vi "Threshold Filter.vi"(11 "Image In":T1) -> (3 "Image Out":T1)   [LabVIEW 2011]
uses:
  <vilib>/vision/Image Controls.llb/IMAQ Image.ctl
  <vilib>/vision/NI_Vision_Development_Module.lvlib
panel:
  in  "Replace Value":i32=1
  out "ThreshHold Filter":T1(plugin-control)
  in  "Blue or Luma or Val or Inten Range":cluster{"Lower value":i32, "Upper value":i32}={"Lower value"=0, "Upper value"=255}
  in  "Green or Sat Range":cluster{"Lower value":i32, "Upper value":i32}={"Lower value"=0, "Upper value"=255}
  in  "Red or Hue Range":cluster{"Lower value":i32, "Upper value":i32}={"Lower value"=0, "Upper value"=255}
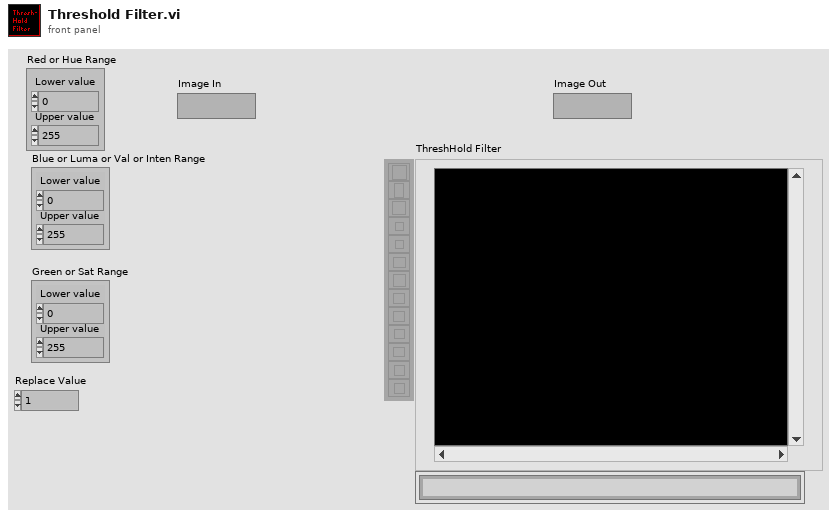
[diagram p1: front panel]
types:
  T1 = typedef "IMAQ Image.ctl" = refnum<image>
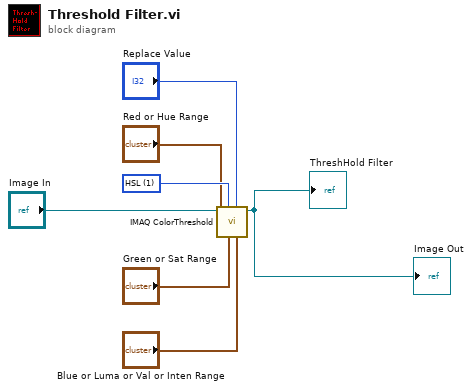
[diagram p0: block diagram]
diagram:
  w7 = u16 1 items=["RGB", "HSL", "HSV", "HSI"] ("Color Mode")
  n1 = call "IMAQ ColorThreshold"("Blue or Luma or Val or Inten Range"="Blue or Luma or Val or Inten Range", "Replace Value"="Replace Value", "Green or Sat Range"="Green or Sat Range", "Color Mode"=w7, "Red or Hue Range"="Red or Hue Range", "Image Src"="Image In") -> ("Image Dst Out"=→"ThreshHold Filter" →"Image Out":T1)  [unwired: 4 in, 1 out]
